vi "LJUD_eDAC.vi"(0 "Handle In":i32, 5 "Channel":i32, 7 "Voltage":dbl format="%.2f", 11 "error in":errorcluster, 12 "Binary":i32) -> (4 "Handle Out":i32, 15 "error out":errorcluster)   [LabVIEW 2017]
doc: "This is an easy function to set the\nvoltage of a single analog output.\n\nSee Sections 4.2 and 4.3 of the device's\ndatasheet for more information."
uses:
  labjackud.dll
panel:
  # "This is an easy function to set the\nvoltage of a single analog output.\n\nSee Sections 4.2 and 4.3 of the device's\ndatasheet for more information."
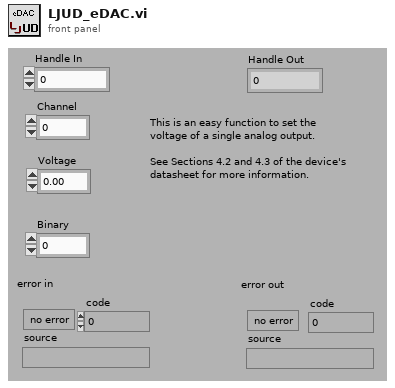
[diagram p1: front panel]
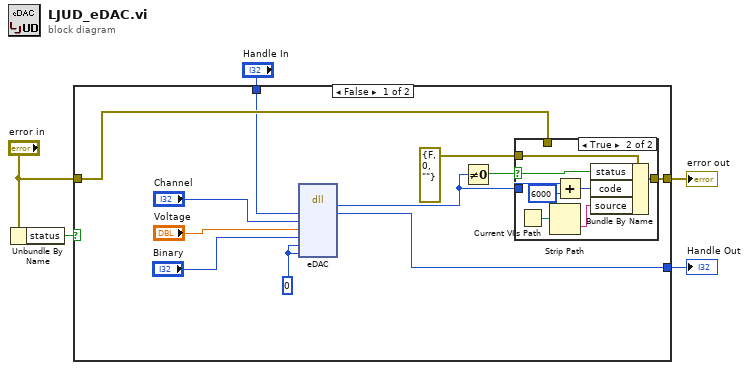
[diagram p0: block diagram]
diagram:
  n1 = Unbundle By Name("error in") -> ("status"=w4:bool)
  n2 = case shown="False" w4 {
    tunnel: [w13 w27] -> w5
    tunnel: "error in" -> [w12 w27]
    tunnel: "Handle In" -> [w7 w26]
    tunnel: [w6 w26] -> w1
    frame False {
      w8 = 0 ("Reserved1")
      n3 = dll-call lib="labjackud.dll" fn="eDAC"("Handle"=w7, "Channel"="Channel", "Voltage"="Voltage", "Binary"="Binary", "Reserved1"=w8, "Reserved2"=w8) -> (w14:i32, "Handle"=w6:i32)  [unwired: 8 in, 2 out]
      n4 = Not Equal To 0?(x=w14) -> (x != 0?=w15:bool)
      n5 = case shown="True" w15 {
        selector: w15 -> [_ w24]
        tunnel: [w17 w25] -> w13
        tunnel: errorcluster {"status"=FALSE, "code"=0, "source"=""} ("error IO") -> [_ w23]
        tunnel: w14 -> [_ w19]
        tunnel: w12 -> [w17 _]
        frame False {
        }
        frame True {
          n6 = Current VI's Path() -> (path=w21:path)
          n7 = Strip Path(path=w21) -> (name=w22:string)  [unwired: 1 out]
          n8 = Add(x=w19, y=6000) -> (x+y=w20:i32)
          n9 = Bundle By Name(cluster=w23, "status"=w24, "code"=w20, "source"=w22) -> (w25:errorcluster)
        }
      }
    }
    frame True {
    }
  }
  "error out" <- w5
  "Handle Out" <- w1
